vi "File_Finder_In-Progress.vi"() -> ()   [LabVIEW 2014]
panel:
  in  "File Directory":path
  in  "Filename":string
  out "Array":bool[][](array[boolean])
  out "filenames":string[](array[string])
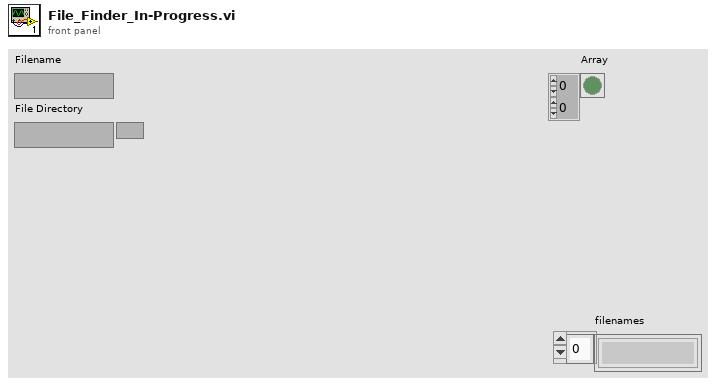
[diagram p1: front panel]
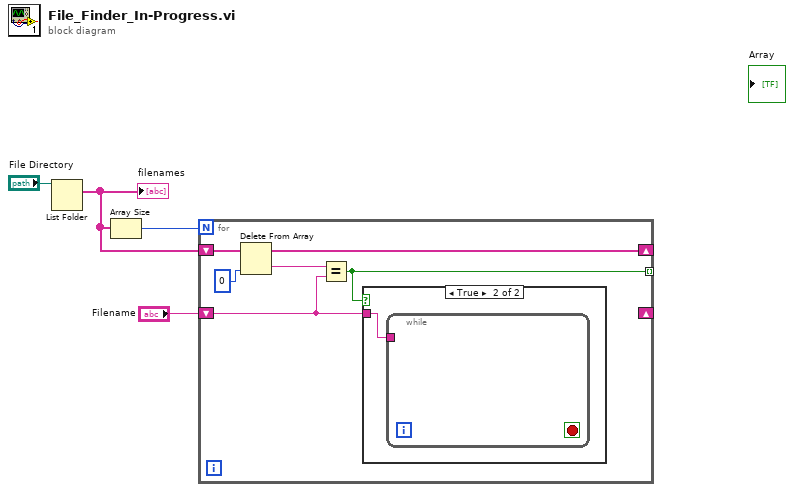
[diagram p0: block diagram]
diagram:
  n1 = List Folder(path="File Directory") -> (filenames=w3:string[])  [unwired: 3 in, 3 out]
  "filenames" <- w3
  n2 = Array Size(array=w3) -> (size(s)=w4:i32)
  n3 = for {
    N: w4 -> [_]
    shift-right: [w8] -> _
    shift-left: w3 -> [w10]
    tunnel: [w6] -> _ mode=indexing
    shift-right: _ -> [_]
    shift-left: "Filename" -> [w5]
    n4 = Delete From Array(array=w10, index=0) -> (deleted portion=w7:string, array with subset deleted=w8:string[])  [unwired: 1 in]
    n5 = Equal?(x=w7, y=w5) -> (x = y?=w6:bool)
    n6 = case shown="True" w6 {
      tunnel: w5 -> [_ w11]
      frame False {
      }
      frame True {
        n7 = while {
          tunnel: w11 -> [_]
          stop <- _ stop-if-true
        }
      }
    }
  }
